vi "Multi-camera acquisition of images.vi"() -> ()   [LabVIEW 2009]
uses:
  D/Program Files (x86)/National Instruments/LabVIEW 2015/user.lib/LabViewDVPCamera/LabViewDVPCamera.lvlib
panel:
  out "new picture 4":picture caption="新图片"
  in  "CloseFlg 4":i32
  in  "CameraList 4":u16(ring) caption="CameraList" items=["USB2_1.2M_MONO(39)@UE121000027", "USB2_3M(19)@1112121"]
  in  "Set 4":bool
  in  "Open 4":bool
  in  "Close 4":bool
  in  "ScanCamera 4":bool
  out "handle 4":u32
  out "new picture 3":picture caption="新图片"
  in  "CloseFlg 3":i32
  in  "CameraList 3":u16(ring) caption="CameraList" items=["USB2_1.2M_MONO(39)@UE121000027", "USB2_3M(19)@1112121"]
  in  "Set 3":bool
  in  "Open 3":bool
  in  "Close 3":bool
  in  "ScanCamera 3":bool
  out "handle 3":u32
  out "new picture 2":picture caption="新图片"
  in  "CloseFlg 2":i32
  in  "CameraList 2":u16(ring) caption="CameraList" items=["USB2_1.2M_MONO(39)@UE121000027", "USB2_3M(19)@1112121"]
  in  "Set 2":bool
  in  "Open 2":bool
  in  "Close 2":bool
  in  "ScanCamera 2":bool
  out "handle 2":u32
  out "new picture":picture caption="新图片"
  in  "CloseFlg":i32
  in  "CameraList":u16(ring) items=["USB2_1.2M_MONO(39)@UE121000027", "USB2_3M(19)@1112121"]
  in  "Set":bool
  in  "Open":bool
  in  "Close":bool
  in  "ScanCamera":bool
  out "handle":u32
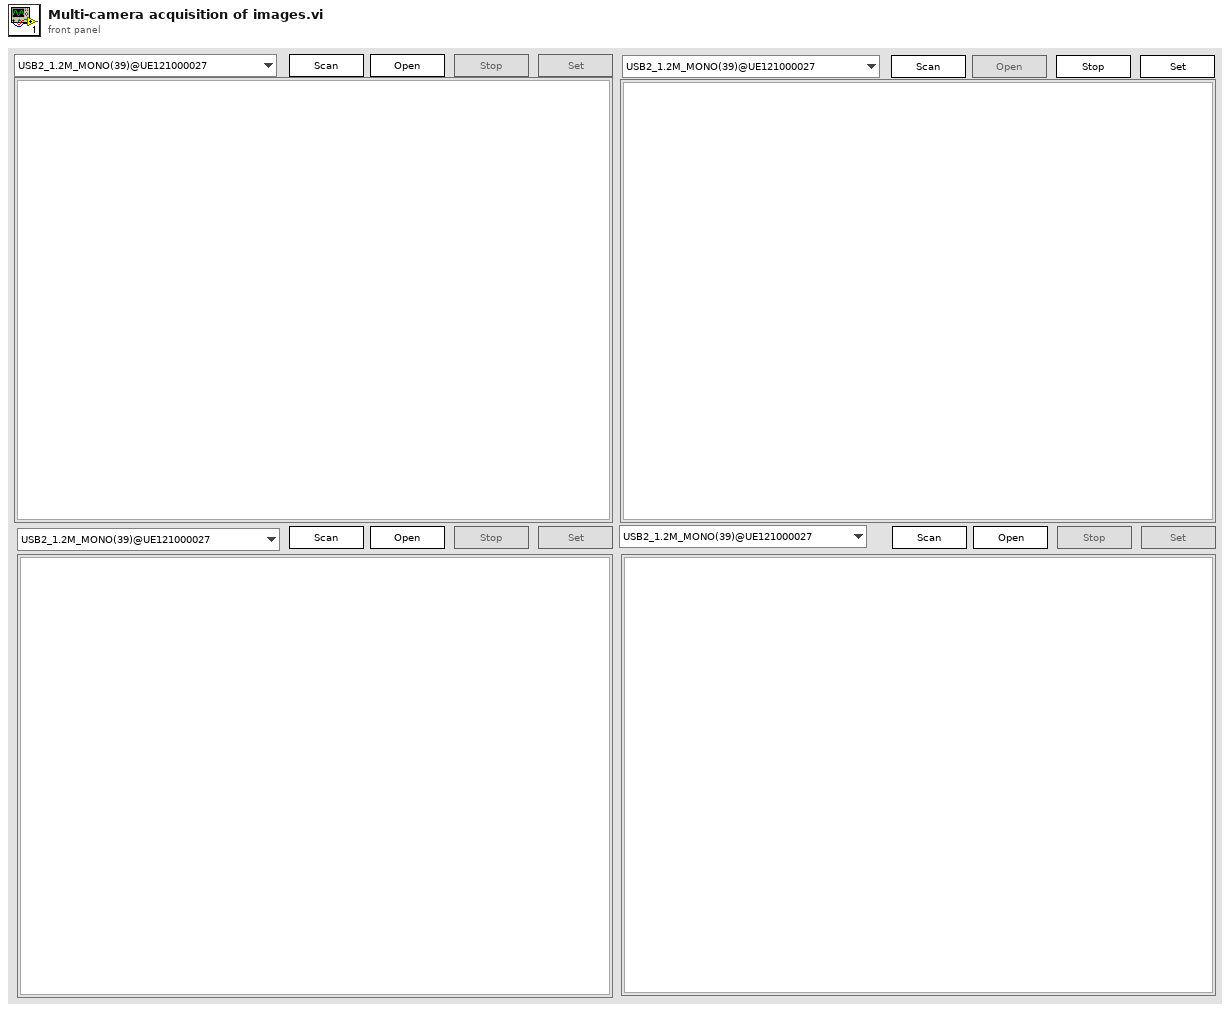
[diagram p1: front panel]
types:
  T1 = enum8{"Enabled", "Disabled", "Disabled and Grayed Out"}
  T2 = typedef "LVStringsAndValuesArrayTypeDef_U16.ctl" = cluster{"String":string, "Value":u16}[]
  T3 = cluster{"image type":i16, "image depth":u8, u8[], "无符号8位数组":u8[], u32[], cluster{u16, u16, u16, u16}}
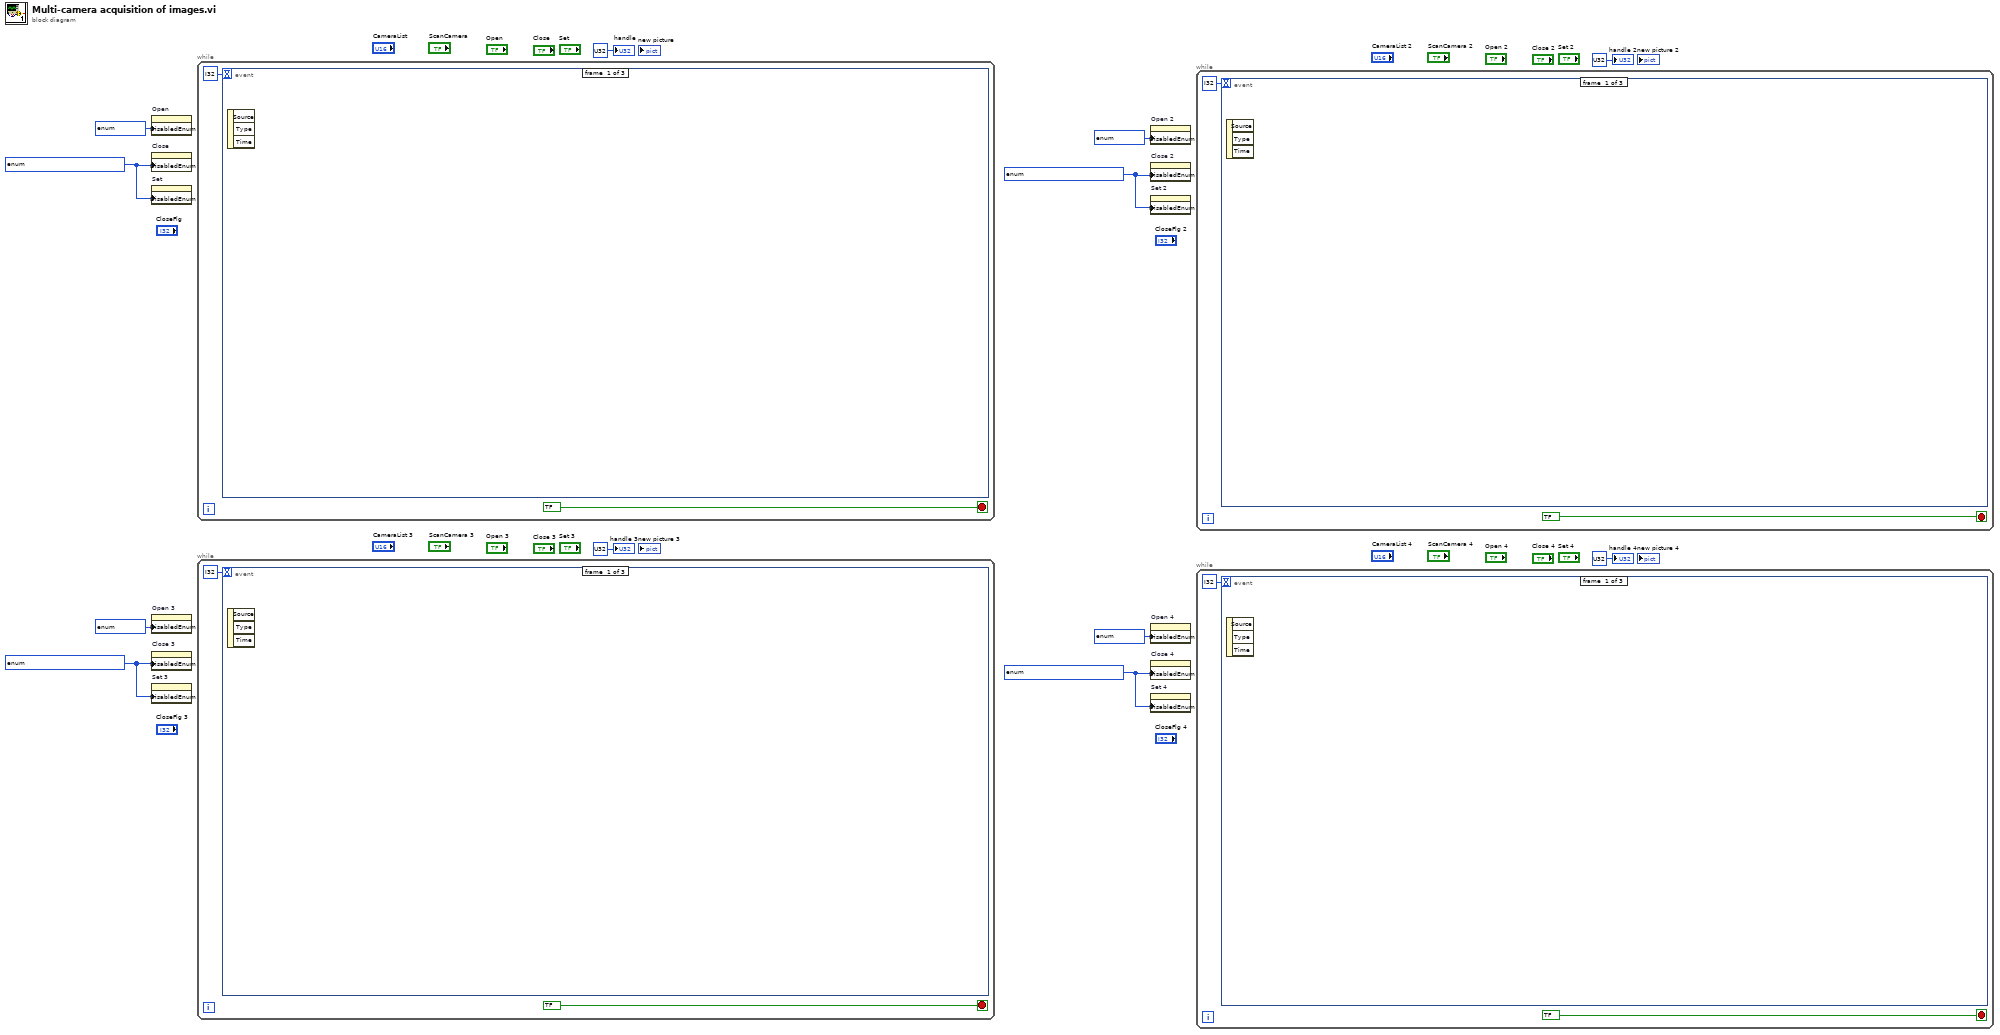
[diagram p0: block diagram]
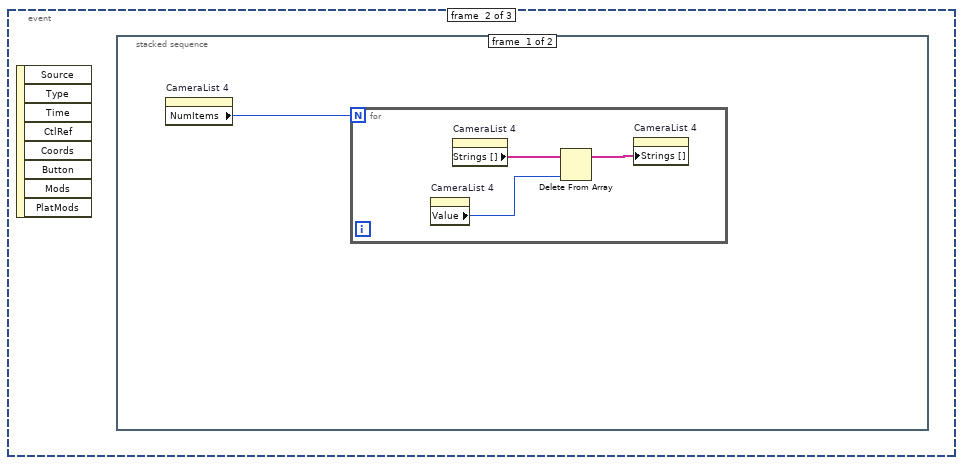
[diagram p2: hidden frame]
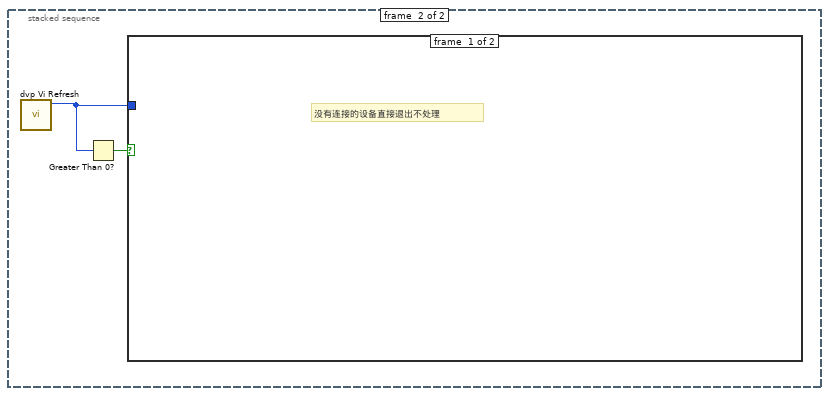
[diagram p3: hidden frame]
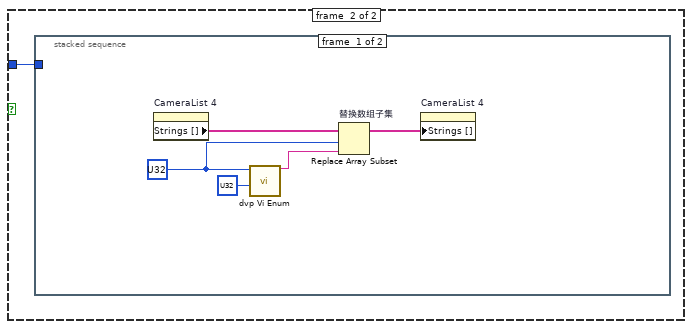
[diagram p4: hidden frame]
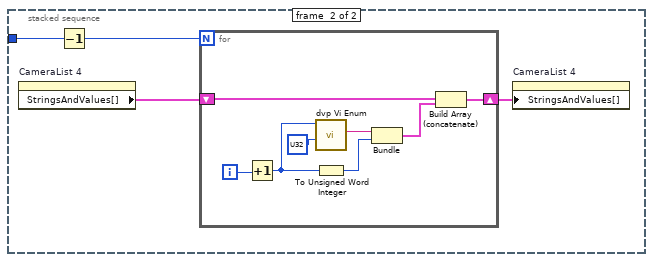
[diagram p5: hidden frame]
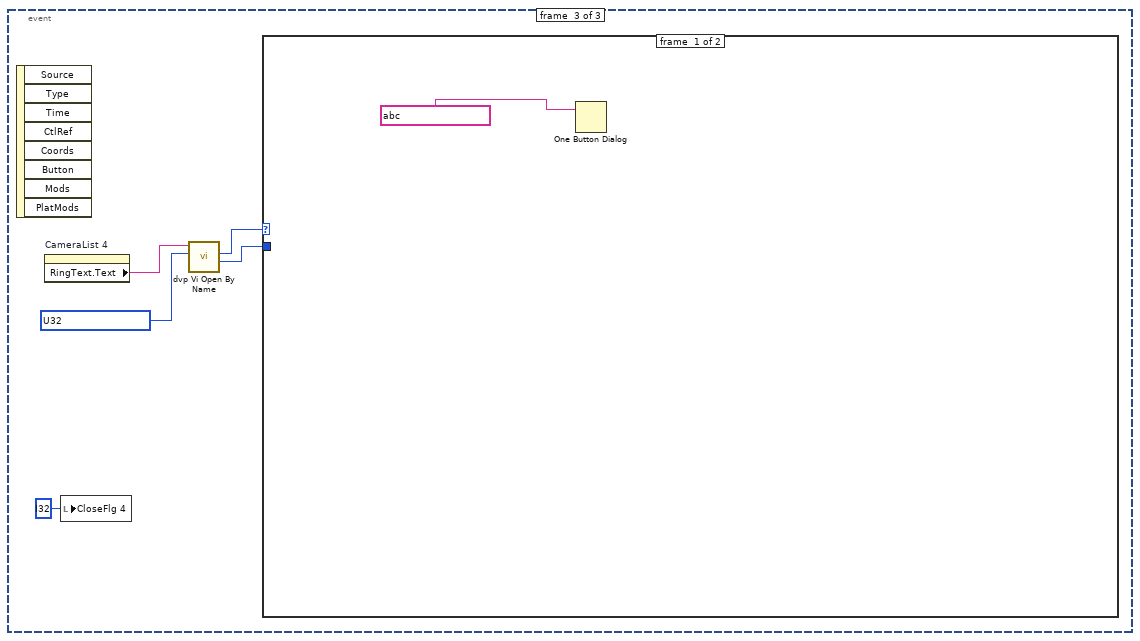
[diagram p6: hidden frame]
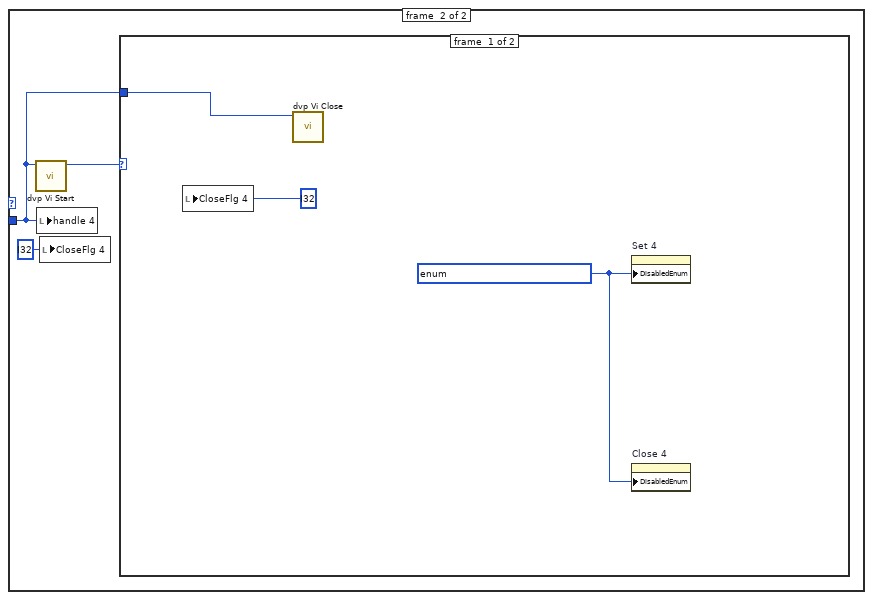
[diagram p7: hidden frame]
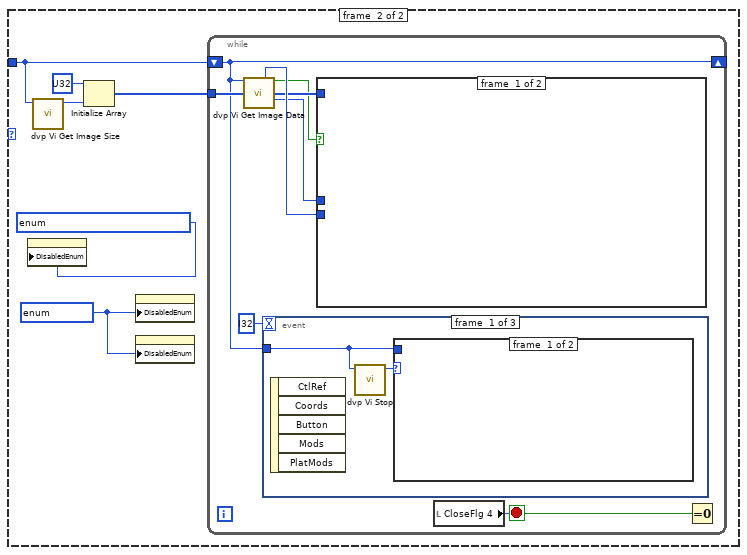
[diagram p8: hidden frame]
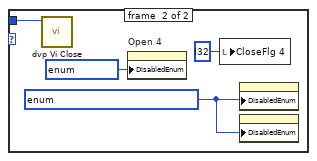
[diagram p9: hidden frame]
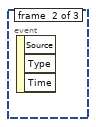
[diagram p10: hidden frame]
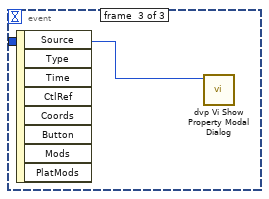
[diagram p11: hidden frame]
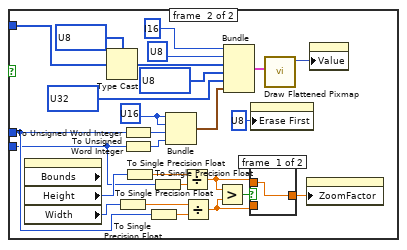
[diagram p12: hidden frame]
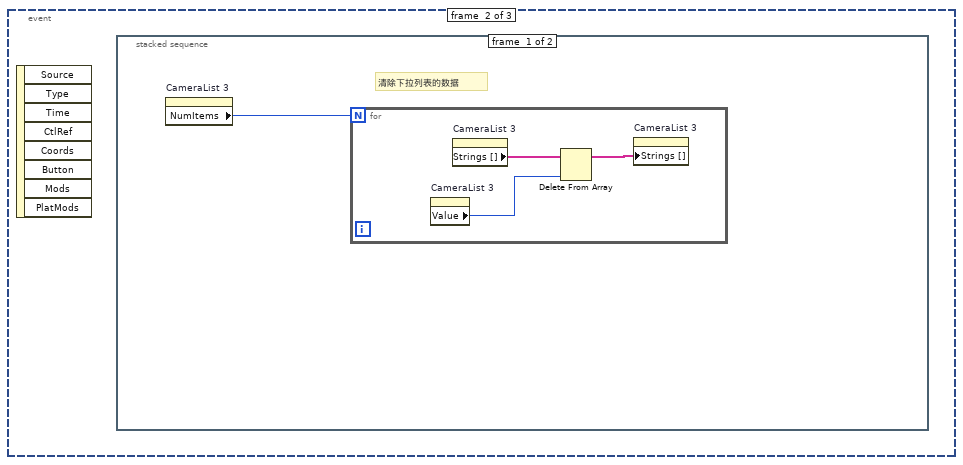
[diagram p14: hidden frame]
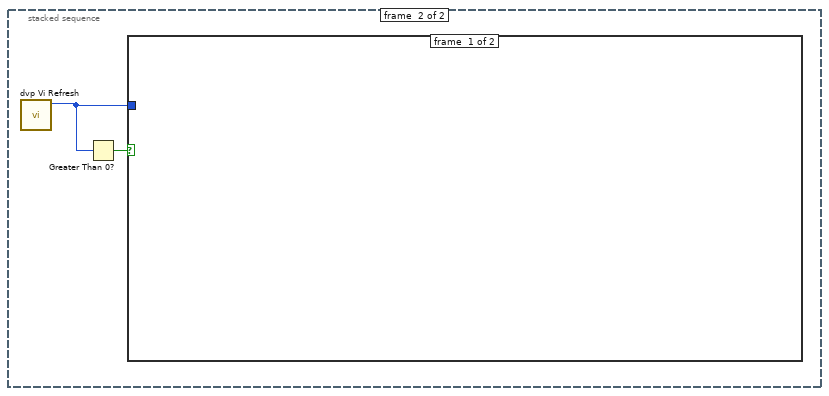
[diagram p15: hidden frame]
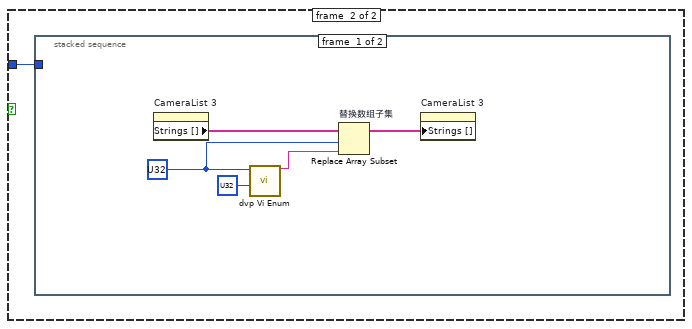
[diagram p16: hidden frame]
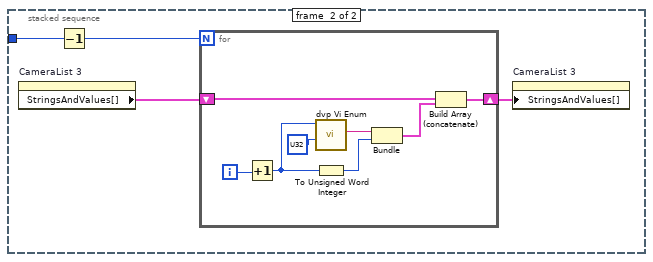
[diagram p17: hidden frame]
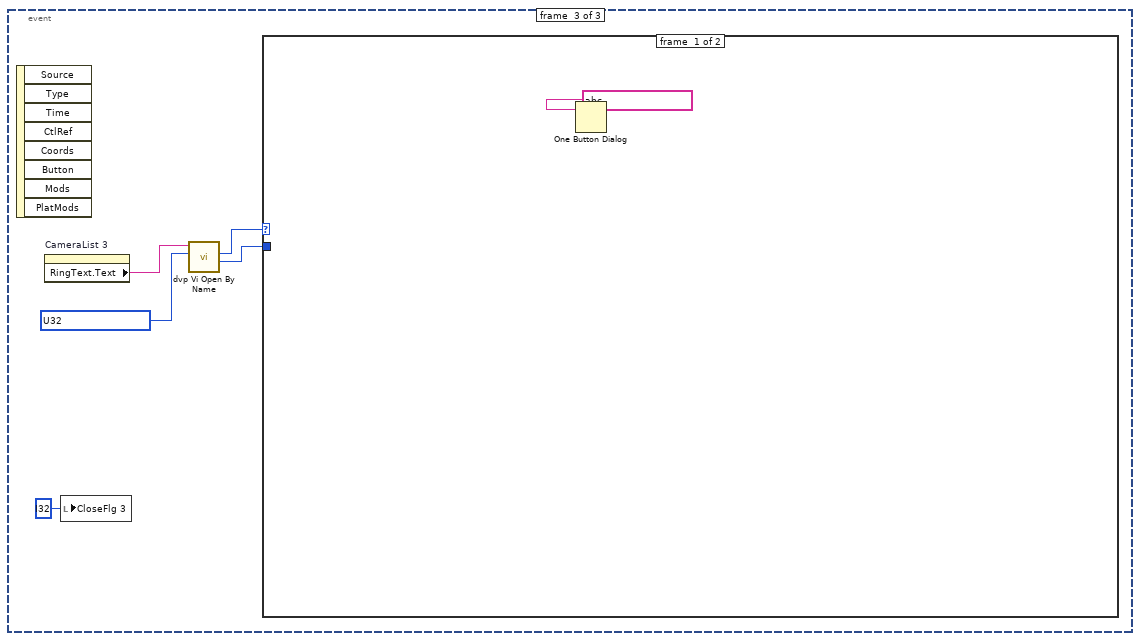
[diagram p18: hidden frame]
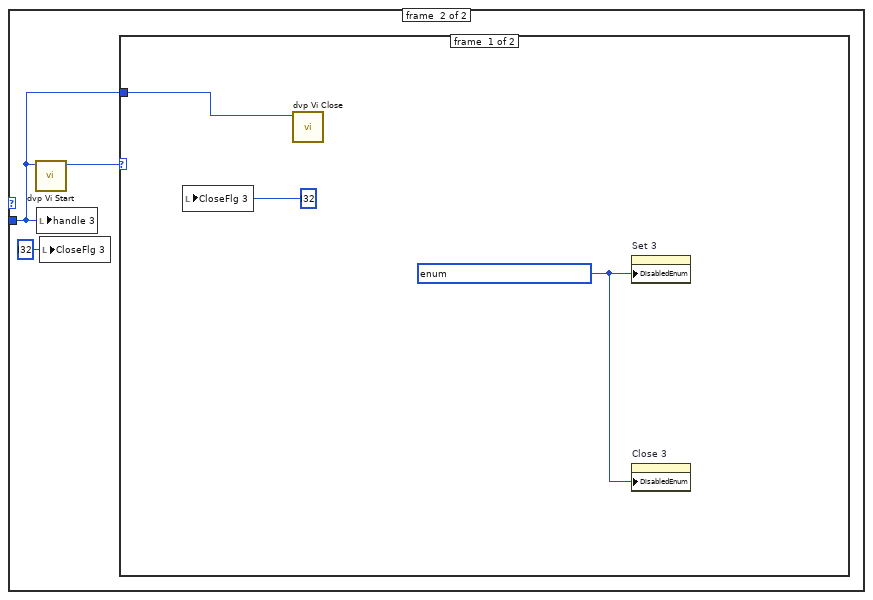
[diagram p19: hidden frame]
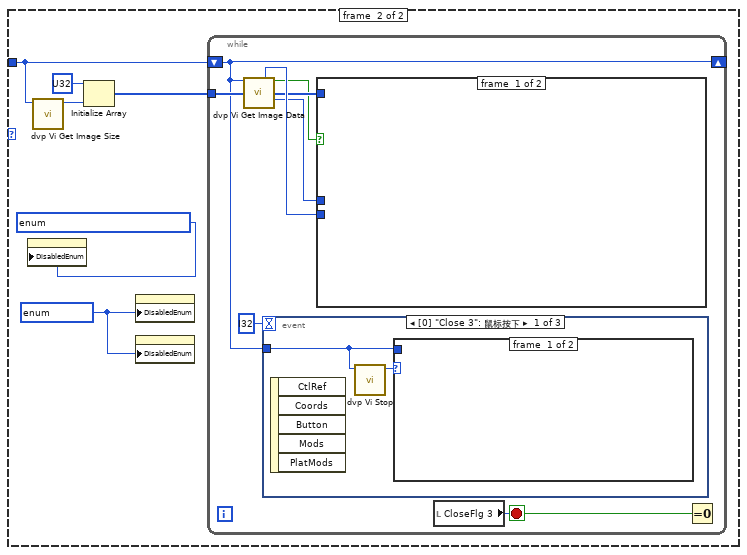
[diagram p20: hidden frame]
diagram:
  w2 = T1 ? ("禁用")
  w5 = T1 ? ("禁用")
  w8 = T1 ? ("禁用")
  w11 = T1 ? ("禁用")
  n1 = property on="Open" class="Bool"("DisabledEnum"=T1 ? ("禁用")) -> ()  [unwired: 2 in, 2 out]
  n2 = property on="Close" class="Bool"("DisabledEnum"=w11) -> ()  [unwired: 2 in, 2 out]
  n3 = property on="Set" class="Bool"("DisabledEnum"=w11) -> ()  [unwired: 2 in, 2 out]
  n4 = property on="Open 3" class="Bool"("DisabledEnum"=T1 ? ("禁用")) -> ()  [unwired: 2 in, 2 out]
  n5 = property on="Close 3" class="Bool"("DisabledEnum"=w5) -> ()  [unwired: 2 in, 2 out]
  n6 = property on="Set 3" class="Bool"("DisabledEnum"=w5) -> ()  [unwired: 2 in, 2 out]
  n7 = while {
    stop <- bool ? stop-if-true
    n8 = event shown="[2] \"Open\": 鼠标按下" {
      selector: _ -> [_ _ _]
      dyn-events: _ -> [_ _ _]
      timeout: i32 ? -> [_ _ _]
      event #0 {
        n9 = event-data() -> ()  [unwired: 1 in, 3 out]
      }
      event #1 {
        n10 = event-data() -> ()  [unwired: 1 in, 8 out]
        n11 = stacked-sequence "清除下拉列表的数据" {
          frame #0 {
            n12 = property on="CameraList" class="Ring (严格)"() -> ("NumItems"=w15:u32)  [unwired: 2 in, 2 out]
            n13 = for {
              N: w15 -> [_]
              n14 = property on="CameraList" class="Ring (严格)"() -> ("Value"=w17:u16)  [unwired: 2 in, 2 out]
              n15 = property on="CameraList" class="Ring (严格)"() -> ("Strings []"=w16:string[])  [unwired: 2 in, 2 out]
              n16 = Delete From Array ("删除数组元素")(array=w16, index=w17) -> (array with subset deleted=w18:string[])  [unwired: 1 in, 1 out]
              n17 = property on="CameraList" class="Ring (严格)"("Strings []"=w18) -> ()  [unwired: 2 in, 2 out]
            }
          }
          frame #1 {
            n18 = call "dvp Vi Refresh.vi"() -> ("pCount out"=w20:u32)  [unwired: 10 in, 1 out]
            n19 = Greater Than 0?(x=w20) -> (x > 0?=w19:bool)
            n20 = case shown="真" w19 {
              tunnel: w20 -> [_ w21]
              frame #0 {
              }
              frame #1 {
                n21 = stacked-sequence {
                  tunnel: w21 -> [_ w28]
                  frame #0 {
                    w22 = u32 ? ("index")
                    n22 = property on="CameraList" class="Ring (严格)"() -> ("Strings []"=w25:string[])  [unwired: 2 in, 2 out]
                    n23 = call "dvp Vi Enum.vi"("unSize"=u32 ?, "index"=w22) -> ("friendlyName out"=w24:string)  [unwired: 8 in, 1 out]
                    n24 = Replace Array Subset "替换数组子集"(array=w25, new element=w24, index=w22) -> (w26:string[])
                    n25 = property on="CameraList" class="Ring (严格)"("Strings []"=w26) -> ()  [unwired: 2 in, 2 out]
                  }
                  frame #1 {
                    n26 = property on="CameraList" class="Ring (严格)"() -> ("StringsAndValues[]"=w30:T2)  [unwired: 2 in, 2 out]
                    n27 = Decrement(x=w28) -> (x-1=w27:u32)
                    n28 = for {
                      N: w27 -> [_]
                      shift-right: [w37] -> w29
                      shift-left: w30 -> [w35]
                      i -> [w32]
                      n29 = Increment(x=w32) -> (x+1=w31:i32)
                      n30 = call "dvp Vi Enum.vi"("unSize"=u32 ?, "index"=w31) -> ("friendlyName out"=w38:string)  [unwired: 8 in, 1 out]
                      n31 = To Unsigned Word Integer(number=w31) -> (unsigned 16bit integer=w34:u16)
                      n32 = Bundle("friendlyName out"=w38, w34) -> (w36:cluster{"friendlyName out":string, u16})  [unwired: 1 in]
                      n33 = Build Array (concatenate)(w35, w36) -> (w37:T2)
                    }
                    n34 = property on="CameraList" class="Ring (严格)"("StringsAndValues[]"=w29) -> ()  [unwired: 2 in, 2 out]
                  }
                }
              }
            }
          }
        }
      }
      event #2 {
        w41 = u32 ? items=["OPEN_OFFLINE", "OPEN_NORMAL"] ("type")
        n35 = event-data() -> ()  [unwired: 1 in, 8 out]
        n36 = property on="CameraList" class="Ring (严格)"() -> ("RingText.Text"=w40:string)  [unwired: 2 in, 2 out]
        n37 = local write "CloseFlg"(i32 ? ("CloseFlg")) -> ()
        n38 = call "dvp Vi Open By Name.vi"("type"=w41, "friendlyName"=w40) -> ("pHandle out"=w43:u32, "function return"=w42:u32)  [unwired: 7 in, 1 out]
        n39 = case shown="1" w42 {
          tunnel: w43 -> [_ w47]
          frame #0 {
            n40 = One Button Dialog(message=string ? ("消息")) -> ()  [unwired: 1 in, 1 out]
          }
          frame #1 {
            n41 = call "dvp Vi Start.vi"("handle"=w47) -> ("function return"=w45:u32)  [unwired: 10 in]
            n42 = local write "handle"(w47) -> ()
            n43 = local write "CloseFlg"(i32 ? ("CloseFlg")) -> ()
            n44 = case shown="1" w45 {
              tunnel: w47 -> [w50 w52]
              frame #0 {
                w49 = T1 ? ("禁用")
                n45 = local write "CloseFlg"(i32 ? ("CloseFlg")) -> ()
                n46 = call "dvp Vi Close.vi"("handle"=w50) -> ()  [unwired: 10 in, 1 out]
                n47 = property on="Set" class="Bool"("DisabledEnum"=w49) -> ()  [unwired: 2 in, 2 out]
                n48 = property on="Close" class="Bool"("DisabledEnum"=w49) -> ()  [unwired: 2 in, 2 out]
              }
              frame #1 {
                w56 = T1 ? ("禁用")
                n49 = property on="Open" class="Bool"("DisabledEnum"=T1 ? ("禁用")) -> ()  [unwired: 2 in, 2 out]
                n50 = call "dvp Vi Get Image Size.vi"("handle"=w52) -> ("function return"=w51:u32)  [unwired: 10 in]
                n51 = Initialize Array(u32 ? ("元素"), w51) -> (w53:u32[])
                n52 = property on="Set" class="Bool"("DisabledEnum"=w56) -> ()  [unwired: 2 in, 2 out]
                n53 = property on="Close" class="Bool"("DisabledEnum"=w56) -> ()  [unwired: 2 in, 2 out]
                n54 = while {
                  shift-right: [w61] -> _
                  shift-left: w52 -> [w61]
                  tunnel: w53 -> [w62]
                  stop <- w64 stop-if-true
                  n55 = call "dvp Vi Get Image Data.vi"("handle"=w61, "pbuffer"=w62) -> ("piHeight out"=w60:i32, "function return"=w57:bool, "pbuffer out"=w58:u32[], "piWidth out"=w59:i32)  [unwired: 9 in, 1 out]
                  n56 = event shown="[0] \"Close\": 鼠标按下" {
                    selector: _ -> [_ _ _]
                    dyn-events: _ -> [_ _ _]
                    timeout: i32 ? -> [_ _ _]
                    tunnel: w61 -> [w66 _ w72]
                    event #0 {
                      n57 = event-data() -> ()  [unwired: 1 in, 5 out]
                      n58 = call "dvp Vi Stop.vi"("handle"=w66) -> ("function return"=w67:u32)  [unwired: 10 in]
                      n59 = case shown="1" w67 {
                        tunnel: w66 -> [_ w69]
                        frame #0 {
                        }
                        frame #1 {
                          w68 = T1 ? ("禁用")
                          n60 = call "dvp Vi Close.vi"("handle"=w69) -> ()  [unwired: 10 in, 1 out]
                          n61 = property on="Open" class="Bool"("DisabledEnum"=T1 ? ("禁用")) -> ()  [unwired: 2 in, 2 out]
                          n62 = local write "CloseFlg"(i32 ? ("CloseFlg")) -> ()
                          n63 = property on="Close" class="Bool"("DisabledEnum"=w68) -> ()  [unwired: 2 in, 2 out]
                          n64 = property on="Set" class="Bool"("DisabledEnum"=w68) -> ()  [unwired: 2 in, 2 out]
                        }
                      }
                    }
                    event #1 {
                      n65 = event-data() -> ()  [unwired: 1 in, 3 out]
                    }
                    event #2 {
                      n66 = event-data() -> ()  [unwired: 1 in, 8 out]
                      n67 = call "dvp Vi Show Property Modal Dialog.vi"("handle"=w72) -> ()  [unwired: 10 in, 1 out]
                    }
                  }
                  n68 = case shown="真" w57 {
                    tunnel: w58 -> [_ w76]
                    tunnel: w59 -> [_ w80]
                    tunnel: w60 -> [_ w79]
                    frame #0 {
                    }
                    frame #1 {
                      w96 = u16 ?
                      n69 = property on="new picture" class="Pict" props=[]() -> ("Height"=w89:u32, "Width"=w88:u32)  [unwired: 2 in, 3 out]
                      n70 = Type Cast(type=u8[] ?, x=w76) -> (*(type *) &x=w75:u8[])
                      n71 = To Single Precision Float(number=w88) -> (single precision float=w81:sgl)
                      n72 = To Unsigned Word Integer(number=w80) -> (unsigned 16bit integer=w95:u16)
                      n73 = To Unsigned Word Integer(number=w79) -> (unsigned 16bit integer=w94:u16)
                      n74 = To Single Precision Float(number=w89) -> (single precision float=w87:sgl)
                      n75 = To Single Precision Float(number=w80) -> (single precision float=w85:sgl)
                      n76 = To Single Precision Float(number=w79) -> (single precision float=w86:sgl)
                      n77 = Bundle ("图像尺寸")(w96, w96, w95, w94) -> (w93:cluster{u16, u16, u16, u16})  [unwired: 1 in]
                      n78 = Divide(x=w87, y=w86) -> (x/y=w83:sgl)
                      n79 = Divide(x=w81, y=w85) -> (x/y=w82:sgl)
                      n80 = Greater?(x=w83, y=w82) -> (0:w84:bool)
                      n81 = Bundle ("图像数据")("image type"=i16 ?, "image depth"=u8 ?, w75, "无符号8位数组"=u8[] ?, u32[] ?, w93) -> (w77:T3)  [unwired: 1 in]
                      n82 = case shown="真" w84 {
                        tunnel: w83 -> [w99 _]
                        tunnel: w82 -> [_ w100]
                        tunnel: [w99 w100] -> w78
                        frame #0 {
                        }
                        frame #1 {
                        }
                      }
                      n83 = property on="new picture" class="Pict"("Erase First"=u8 ? ("画前清除图片")) -> ()  [unwired: 2 in, 2 out]
                      n84 = call <vilib>:"Draw Flattened Pixmap.vi"("image data"=w77) -> ("new picture"=w90:picture)  [unwired: 8 in]
                      n85 = property on="new picture" class="Pict"("ZoomFactor"=w78) -> ()  [unwired: 2 in, 2 out]
                      n86 = property on="new picture" class="Pict"("Value"=w90) -> ()  [unwired: 2 in, 2 out]
                    }
                  }
                  n87 = local read "CloseFlg"() -> (w63:i32)
                  n88 = Equal To 0?(x=w63) -> (x = 0?=w64:bool)
                }
              }
            }
          }
        }
      }
    }
  }
  n89 = while {
    stop <- bool ? stop-if-true
    n90 = event shown="[2] \"Open 3\": 鼠标按下" {
      selector: _ -> [_ _ _]
      dyn-events: _ -> [_ _ _]
      timeout: i32 ? -> [_ _ _]
      event #0 {
        n91 = event-data() -> ()  [unwired: 1 in, 3 out]
      }
      event #1 {
        n92 = event-data() -> ()  [unwired: 1 in, 8 out]
        n93 = stacked-sequence "清除下拉列表的数据" {
          frame #0 {
            # "清除下拉列表的数据"
            n94 = property on="CameraList 3" class="Ring (严格)"() -> ("NumItems"=w103:u32)  [unwired: 2 in, 2 out]
            n95 = for {
              N: w103 -> [_]
              n96 = property on="CameraList 3" class="Ring (严格)"() -> ("Value"=w105:u16)  [unwired: 2 in, 2 out]
              n97 = property on="CameraList 3" class="Ring (严格)"() -> ("Strings []"=w104:string[])  [unwired: 2 in, 2 out]
              n98 = Delete From Array ("删除数组元素")(array=w104, index=w105) -> (array with subset deleted=w106:string[])  [unwired: 1 in, 1 out]
              n99 = property on="CameraList 3" class="Ring (严格)"("Strings []"=w106) -> ()  [unwired: 2 in, 2 out]
            }
          }
          frame #1 {
            n100 = call "dvp Vi Refresh.vi"() -> ("pCount out"=w108:u32)  [unwired: 10 in, 1 out]
            n101 = Greater Than 0?(x=w108) -> (x > 0?=w107:bool)
            n102 = case shown="真" w107 {
              tunnel: w108 -> [_ w109]
              frame #0 {
              }
              frame #1 {
                n103 = stacked-sequence {
                  tunnel: w109 -> [_ w116]
                  frame #0 {
                    w110 = u32 ? ("index")
                    n104 = property on="CameraList 3" class="Ring (严格)"() -> ("Strings []"=w113:string[])  [unwired: 2 in, 2 out]
                    n105 = call "dvp Vi Enum.vi"("unSize"=u32 ?, "index"=w110) -> ("friendlyName out"=w112:string)  [unwired: 8 in, 1 out]
                    n106 = Replace Array Subset "替换数组子集"(array=w113, new element=w112, index=w110) -> (w114:string[])
                    n107 = property on="CameraList 3" class="Ring (严格)"("Strings []"=w114) -> ()  [unwired: 2 in, 2 out]
                  }
                  frame #1 {
                    n108 = property on="CameraList 3" class="Ring (严格)"() -> ("StringsAndValues[]"=w118:T2)  [unwired: 2 in, 2 out]
                    n109 = Decrement(x=w116) -> (x-1=w115:u32)
                    n110 = for {
                      N: w115 -> [_]
                      shift-right: [w125] -> w117
                      shift-left: w118 -> [w123]
                      i -> [w120]
                      n111 = Increment(x=w120) -> (x+1=w119:i32)
                      n112 = call "dvp Vi Enum.vi"("unSize"=u32 ?, "index"=w119) -> ("friendlyName out"=w126:string)  [unwired: 8 in, 1 out]
                      n113 = To Unsigned Word Integer(number=w119) -> (unsigned 16bit integer=w122:u16)
                      n114 = Bundle("friendlyName out"=w126, w122) -> (w124:cluster{"friendlyName out":string, u16})  [unwired: 1 in]
                      n115 = Build Array (concatenate)(w123, w124) -> (w125:T2)
                    }
                    n116 = property on="CameraList 3" class="Ring (严格)"("StringsAndValues[]"=w117) -> ()  [unwired: 2 in, 2 out]
                  }
                }
              }
            }
          }
        }
      }
      event #2 {
        w129 = u32 ? items=["OPEN_OFFLINE", "OPEN_NORMAL"] ("type")
        n117 = event-data() -> ()  [unwired: 1 in, 8 out]
        n118 = property on="CameraList 3" class="Ring (严格)"() -> ("RingText.Text"=w128:string)  [unwired: 2 in, 2 out]
        n119 = local write "CloseFlg 3"(i32 ? ("CloseFlg")) -> ()
        n120 = call "dvp Vi Open By Name.vi"("type"=w129, "friendlyName"=w128) -> ("pHandle out"=w131:u32, "function return"=w130:u32)  [unwired: 7 in, 1 out]
        n121 = case shown="1" w130 {
          tunnel: w131 -> [_ w135]
          frame #0 {
            n122 = One Button Dialog(message=string ? ("消息")) -> ()  [unwired: 1 in, 1 out]
          }
          frame #1 {
            n123 = call "dvp Vi Start.vi"("handle"=w135) -> ("function return"=w133:u32)  [unwired: 10 in]
            n124 = local write "handle 3"(w135) -> ()
            n125 = local write "CloseFlg 3"(i32 ? ("CloseFlg")) -> ()
            n126 = case shown="1" w133 {
              tunnel: w135 -> [w138 w140]
              frame #0 {
                w137 = T1 ? ("禁用")
                n127 = local write "CloseFlg 3"(i32 ? ("CloseFlg")) -> ()
                n128 = call "dvp Vi Close.vi"("handle"=w138) -> ()  [unwired: 10 in, 1 out]
                n129 = property on="Set 3" class="Bool"("DisabledEnum"=w137) -> ()  [unwired: 2 in, 2 out]
                n130 = property on="Close 3" class="Bool"("DisabledEnum"=w137) -> ()  [unwired: 2 in, 2 out]
              }
              frame #1 {
                w144 = T1 ? ("禁用")
                n131 = property on="Open 3" class="Bool"("DisabledEnum"=T1 ? ("禁用")) -> ()  [unwired: 2 in, 2 out]
                n132 = call "dvp Vi Get Image Size.vi"("handle"=w140) -> ("function return"=w139:u32)  [unwired: 10 in]
                n133 = Initialize Array(u32 ? ("元素"), w139) -> (w141:u32[])
                n134 = property on="Set 3" class="Bool"("DisabledEnum"=w144) -> ()  [unwired: 2 in, 2 out]
                n135 = property on="Close 3" class="Bool"("DisabledEnum"=w144) -> ()  [unwired: 2 in, 2 out]
                n136 = while {
                  shift-right: [w149] -> _
                  shift-left: w140 -> [w149]
                  tunnel: w141 -> [w150]
                  stop <- w152 stop-if-true
                  n137 = call "dvp Vi Get Image Data.vi"("handle"=w149, "pbuffer"=w150) -> ("piHeight out"=w148:i32, "function return"=w145:bool, "pbuffer out"=w146:u32[], "piWidth out"=w147:i32)  [unwired: 9 in, 1 out]
                  n138 = event shown="[0] \"Close 3\": 鼠标按下" {
                    selector: _ -> [_ _ _]
                    dyn-events: _ -> [_ _ _]
                    timeout: i32 ? -> [_ _ _]
                    tunnel: w149 -> [w154 _ w160]
                    event #0 {
                      n139 = event-data() -> ()  [unwired: 1 in, 5 out]
                      n140 = call "dvp Vi Stop.vi"("handle"=w154) -> ("function return"=w155:u32)  [unwired: 10 in]
                      n141 = case shown="1" w155 {
                        tunnel: w154 -> [_ w157]
                        frame #0 {
                        }
                        frame #1 {
                          w156 = T1 ? ("禁用")
                          n142 = call "dvp Vi Close.vi"("handle"=w157) -> ()  [unwired: 10 in, 1 out]
                          n143 = property on="Open 3" class="Bool"("DisabledEnum"=T1 ? ("禁用")) -> ()  [unwired: 2 in, 2 out]
                          n144 = local write "CloseFlg 3"(i32 ? ("CloseFlg")) -> ()
                          n145 = property on="Close 3" class="Bool"("DisabledEnum"=w156) -> ()  [unwired: 2 in, 2 out]
                          n146 = property on="Set 3" class="Bool"("DisabledEnum"=w156) -> ()  [unwired: 2 in, 2 out]
                        }
                      }
                    }
                    event #1 {
                      n147 = event-data() -> ()  [unwired: 1 in, 3 out]
                    }
                    event #2 {
                      n148 = event-data() -> ()  [unwired: 1 in, 8 out]
                      n149 = call "dvp Vi Show Property Modal Dialog.vi"("handle"=w160) -> ()  [unwired: 10 in, 1 out]
                    }
                  }
                  n150 = case shown="真" w145 {
                    tunnel: w146 -> [_ w164]
                    tunnel: w147 -> [_ w168]
                    tunnel: w148 -> [_ w167]
                    frame #0 {
                    }
                    frame #1 {
                      w184 = u16 ?
                      n151 = property on="new picture 3" class="Pict" props=[]() -> ("Height"=w177:u32, "Width"=w176:u32)  [unwired: 2 in, 3 out]
                      n152 = Type Cast(type=u8[] ?, x=w164) -> (*(type *) &x=w163:u8[])
                      n153 = To Single Precision Float(number=w176) -> (single precision float=w169:sgl)
                      n154 = To Unsigned Word Integer(number=w168) -> (unsigned 16bit integer=w183:u16)
                      n155 = To Unsigned Word Integer(number=w167) -> (unsigned 16bit integer=w182:u16)
                      n156 = To Single Precision Float(number=w177) -> (single precision float=w175:sgl)
                      n157 = To Single Precision Float(number=w168) -> (single precision float=w173:sgl)
                      n158 = To Single Precision Float(number=w167) -> (single precision float=w174:sgl)
                      n159 = Bundle ("图像尺寸")(w184, w184, w183, w182) -> (w181:cluster{u16, u16, u16, u16})  [unwired: 1 in]
                      n160 = Divide(x=w175, y=w174) -> (x/y=w171:sgl)
                      n161 = Divide(x=w169, y=w173) -> (x/y=w170:sgl)
                      n162 = Greater?(x=w171, y=w170) -> (0:w172:bool)
                      n163 = Bundle ("图像数据")("image type"=i16 ?, "image depth"=u8 ?, w163, "无符号8位数组"=u8[] ?, u32[] ?, w181) -> (w165:T3)  [unwired: 1 in]
                      n164 = case shown="真" w172 {
                        tunnel: w171 -> [w187 _]
                        tunnel: w170 -> [_ w188]
                        tunnel: [w187 w188] -> w166
                        frame #0 {
                        }
                        frame #1 {
                        }
                      }
                      n165 = property on="new picture 3" class="Pict"("Erase First"=u8 ? ("画前清除图片")) -> ()  [unwired: 2 in, 2 out]
                      n166 = call <vilib>:"Draw Flattened Pixmap.vi"("image data"=w165) -> ("new picture"=w178:picture)  [unwired: 8 in]
                      n167 = property on="new picture 3" class="Pict"("ZoomFactor"=w166) -> ()  [unwired: 2 in, 2 out]
                      n168 = property on="new picture 3" class="Pict"("Value"=w178) -> ()  [unwired: 2 in, 2 out]
                    }
                  }
                  n169 = local read "CloseFlg 3"() -> (w151:i32)
                  n170 = Equal To 0?(x=w151) -> (x = 0?=w152:bool)
                }
              }
            }
          }
        }
      }
    }
  }
  n171 = property on="Open 2" class="Bool"("DisabledEnum"=T1 ? ("禁用")) -> ()  [unwired: 2 in, 2 out]
  n172 = property on="Close 2" class="Bool"("DisabledEnum"=w8) -> ()  [unwired: 2 in, 2 out]
  n173 = property on="Set 2" class="Bool"("DisabledEnum"=w8) -> ()  [unwired: 2 in, 2 out]
  n174 = property on="Open 4" class="Bool"("DisabledEnum"=T1 ? ("禁用")) -> ()  [unwired: 2 in, 2 out]
  n175 = property on="Close 4" class="Bool"("DisabledEnum"=w2) -> ()  [unwired: 2 in, 2 out]
  n176 = property on="Set 4" class="Bool"("DisabledEnum"=w2) -> ()  [unwired: 2 in, 2 out]
  n177 = while {
    stop <- bool ? stop-if-true
    n178 = event shown="[2] \"Open 2\": 鼠标按下" {
      selector: _ -> [_ _ _]
      dyn-events: _ -> [_ _ _]
      timeout: i32 ? -> [_ _ _]
      event #0 {
        n179 = event-data() -> ()  [unwired: 1 in, 3 out]
      }
      event #1 {
        n180 = event-data() -> ()  [unwired: 1 in, 8 out]
        n181 = stacked-sequence "清除下拉列表的数据" {
          frame #0 {
            n182 = property on="CameraList 2" class="Ring (严格)"() -> ("NumItems"=w191:u32)  [unwired: 2 in, 2 out]
            n183 = for {
              N: w191 -> [_]
              n184 = property on="CameraList 2" class="Ring (严格)"() -> ("Value"=w193:u16)  [unwired: 2 in, 2 out]
              n185 = property on="CameraList 2" class="Ring (严格)"() -> ("Strings []"=w192:string[])  [unwired: 2 in, 2 out]
              n186 = Delete From Array ("删除数组元素")(array=w192, index=w193) -> (array with subset deleted=w194:string[])  [unwired: 1 in, 1 out]
              n187 = property on="CameraList 2" class="Ring (严格)"("Strings []"=w194) -> ()  [unwired: 2 in, 2 out]
            }
          }
          frame #1 {
            n188 = call "dvp Vi Refresh.vi"() -> ("pCount out"=w196:u32)  [unwired: 10 in, 1 out]
            n189 = Greater Than 0?(x=w196) -> (x > 0?=w195:bool)
            n190 = case shown="真" w195 {
              tunnel: w196 -> [_ w197]
              frame #0 {
              }
              frame #1 {
                n191 = stacked-sequence {
                  tunnel: w197 -> [_ w204]
                  frame #0 {
                    w198 = u32 ? ("index")
                    n192 = property on="CameraList 2" class="Ring (严格)"() -> ("Strings []"=w201:string[])  [unwired: 2 in, 2 out]
                    n193 = call "dvp Vi Enum.vi"("unSize"=u32 ?, "index"=w198) -> ("friendlyName out"=w200:string)  [unwired: 8 in, 1 out]
                    n194 = Replace Array Subset "替换数组子集"(array=w201, new element=w200, index=w198) -> (w202:string[])
                    n195 = property on="CameraList 2" class="Ring (严格)"("Strings []"=w202) -> ()  [unwired: 2 in, 2 out]
                  }
                  frame #1 {
                    n196 = property on="CameraList 2" class="Ring (严格)"() -> ("StringsAndValues[]"=w206:T2)  [unwired: 2 in, 2 out]
                    n197 = Decrement(x=w204) -> (x-1=w203:u32)
                    n198 = for {
                      N: w203 -> [_]
                      shift-right: [w213] -> w205
                      shift-left: w206 -> [w211]
                      i -> [w208]
                      n199 = Increment(x=w208) -> (x+1=w207:i32)
                      n200 = call "dvp Vi Enum.vi"("unSize"=u32 ?, "index"=w207) -> ("friendlyName out"=w214:string)  [unwired: 8 in, 1 out]
                      n201 = To Unsigned Word Integer(number=w207) -> (unsigned 16bit integer=w210:u16)
                      n202 = Bundle("friendlyName out"=w214, w210) -> (w212:cluster{"friendlyName out":string, u16})  [unwired: 1 in]
                      n203 = Build Array (concatenate)(w211, w212) -> (w213:T2)
                    }
                    n204 = property on="CameraList 2" class="Ring (严格)"("StringsAndValues[]"=w205) -> ()  [unwired: 2 in, 2 out]
                  }
                }
              }
            }
          }
        }
      }
      event #2 {
        w217 = u32 ? items=["OPEN_OFFLINE", "OPEN_NORMAL"] ("type")
        n205 = event-data() -> ()  [unwired: 1 in, 8 out]
        n206 = property on="CameraList 2" class="Ring (严格)"() -> ("RingText.Text"=w216:string)  [unwired: 2 in, 2 out]
        n207 = local write "CloseFlg 2"(i32 ? ("CloseFlg")) -> ()
        n208 = call "dvp Vi Open By Name.vi"("type"=w217, "friendlyName"=w216) -> ("pHandle out"=w219:u32, "function return"=w218:u32)  [unwired: 7 in, 1 out]
        n209 = case shown="1" w218 {
          tunnel: w219 -> [_ w223]
          frame #0 {
            n210 = One Button Dialog(message=string ? ("消息")) -> ()  [unwired: 1 in, 1 out]
          }
          frame #1 {
            n211 = call "dvp Vi Start.vi"("handle"=w223) -> ("function return"=w221:u32)  [unwired: 10 in]
            n212 = local write "handle 2"(w223) -> ()
            n213 = local write "CloseFlg 2"(i32 ? ("CloseFlg")) -> ()
            n214 = case shown="1" w221 {
              tunnel: w223 -> [w226 w228]
              frame #0 {
                w225 = T1 ? ("禁用")
                n215 = local write "CloseFlg 2"(i32 ? ("CloseFlg")) -> ()
                n216 = call "dvp Vi Close.vi"("handle"=w226) -> ()  [unwired: 10 in, 1 out]
                n217 = property on="Set 2" class="Bool"("DisabledEnum"=w225) -> ()  [unwired: 2 in, 2 out]
                n218 = property on="Close 2" class="Bool"("DisabledEnum"=w225) -> ()  [unwired: 2 in, 2 out]
              }
              frame #1 {
                w232 = T1 ? ("禁用")
                n219 = property on="Open 2" class="Bool"("DisabledEnum"=T1 ? ("禁用")) -> ()  [unwired: 2 in, 2 out]
                n220 = call "dvp Vi Get Image Size.vi"("handle"=w228) -> ("function return"=w227:u32)  [unwired: 10 in]
                n221 = Initialize Array(u32 ? ("元素"), w227) -> (w229:u32[])
                n222 = property on="Set 2" class="Bool"("DisabledEnum"=w232) -> ()  [unwired: 2 in, 2 out]
                n223 = property on="Close 2" class="Bool"("DisabledEnum"=w232) -> ()  [unwired: 2 in, 2 out]
                n224 = while {
                  shift-right: [w237] -> _
                  shift-left: w228 -> [w237]
                  tunnel: w229 -> [w238]
                  stop <- w240 stop-if-true
                  n225 = call "dvp Vi Get Image Data.vi"("handle"=w237, "pbuffer"=w238) -> ("piHeight out"=w236:i32, "function return"=w233:bool, "pbuffer out"=w234:u32[], "piWidth out"=w235:i32)  [unwired: 9 in, 1 out]
                  n226 = event shown="[0] \"Close 2\": 鼠标按下" {
                    selector: _ -> [_ _ _]
                    dyn-events: _ -> [_ _ _]
                    timeout: i32 ? -> [_ _ _]
                    tunnel: w237 -> [w242 _ w248]
                    event #0 {
                      n227 = event-data() -> ()  [unwired: 1 in, 5 out]
                      n228 = call "dvp Vi Stop.vi"("handle"=w242) -> ("function return"=w243:u32)  [unwired: 10 in]
                      n229 = case shown="1" w243 {
                        tunnel: w242 -> [_ w245]
                        frame #0 {
                        }
                        frame #1 {
                          w244 = T1 ? ("禁用")
                          n230 = call "dvp Vi Close.vi"("handle"=w245) -> ()  [unwired: 10 in, 1 out]
                          n231 = property on="Open 2" class="Bool"("DisabledEnum"=T1 ? ("禁用")) -> ()  [unwired: 2 in, 2 out]
                          n232 = local write "CloseFlg 2"(i32 ? ("CloseFlg")) -> ()
                          n233 = property on="Close 2" class="Bool"("DisabledEnum"=w244) -> ()  [unwired: 2 in, 2 out]
                          n234 = property on="Set 2" class="Bool"("DisabledEnum"=w244) -> ()  [unwired: 2 in, 2 out]
                        }
                      }
                    }
                    event #1 {
                      n235 = event-data() -> ()  [unwired: 1 in, 3 out]
                    }
                    event #2 {
                      n236 = event-data() -> ()  [unwired: 1 in, 8 out]
                      n237 = call "dvp Vi Show Property Modal Dialog.vi"("handle"=w248) -> ()  [unwired: 10 in, 1 out]
                    }
                  }
                  n238 = case shown="真" w233 {
                    tunnel: w234 -> [_ w252]
                    tunnel: w235 -> [_ w256]
                    tunnel: w236 -> [_ w255]
                    frame #0 {
                    }
                    frame #1 {
                      w272 = u16 ?
                      n239 = property on="new picture 2" class="Pict" props=[]() -> ("Height"=w265:u32, "Width"=w264:u32)  [unwired: 2 in, 3 out]
                      n240 = Type Cast(type=u8[] ?, x=w252) -> (*(type *) &x=w251:u8[])
                      n241 = To Single Precision Float(number=w264) -> (single precision float=w257:sgl)
                      n242 = To Unsigned Word Integer(number=w256) -> (unsigned 16bit integer=w271:u16)
                      n243 = To Unsigned Word Integer(number=w255) -> (unsigned 16bit integer=w270:u16)
                      n244 = To Single Precision Float(number=w265) -> (single precision float=w263:sgl)
                      n245 = To Single Precision Float(number=w256) -> (single precision float=w261:sgl)
                      n246 = To Single Precision Float(number=w255) -> (single precision float=w262:sgl)
                      n247 = Bundle ("图像尺寸")(w272, w272, w271, w270) -> (w269:cluster{u16, u16, u16, u16})  [unwired: 1 in]
                      n248 = Divide(x=w263, y=w262) -> (x/y=w259:sgl)
                      n249 = Divide(x=w257, y=w261) -> (x/y=w258:sgl)
                      n250 = Greater?(x=w259, y=w258) -> (0:w260:bool)
                      n251 = Bundle ("图像数据")("image type"=i16 ?, "image depth"=u8 ?, w251, "无符号8位数组"=u8[] ?, u32[] ?, w269) -> (w253:T3)  [unwired: 1 in]
                      n252 = case shown="真" w260 {
                        tunnel: w259 -> [w275 _]
                        tunnel: w258 -> [_ w276]
                        tunnel: [w275 w276] -> w254
                        frame #0 {
                        }
                        frame #1 {
                        }
                      }
                      n253 = property on="new picture 2" class="Pict"("Erase First"=u8 ? ("画前清除图片")) -> ()  [unwired: 2 in, 2 out]
                      n254 = call <vilib>:"Draw Flattened Pixmap.vi"("image data"=w253) -> ("new picture"=w266:picture)  [unwired: 8 in]
                      n255 = property on="new picture 2" class="Pict"("ZoomFactor"=w254) -> ()  [unwired: 2 in, 2 out]
                      n256 = property on="new picture 2" class="Pict"("Value"=w266) -> ()  [unwired: 2 in, 2 out]
                    }
                  }
                  n257 = local read "CloseFlg 2"() -> (w239:i32)
                  n258 = Equal To 0?(x=w239) -> (x = 0?=w240:bool)
                }
              }
            }
          }
        }
      }
    }
  }
  n259 = while {
    stop <- bool ? stop-if-true
    n260 = event shown="[2] \"Open 4\": 鼠标按下" {
      selector: _ -> [_ _ _]
      dyn-events: _ -> [_ _ _]
      timeout: i32 ? -> [_ _ _]
      event #0 {
        n261 = event-data() -> ()  [unwired: 1 in, 3 out]
      }
      event #1 {
        n262 = event-data() -> ()  [unwired: 1 in, 8 out]
        n263 = stacked-sequence "清除下拉列表的数据" {
          frame #0 {
            n264 = property on="CameraList 4" class="Ring (严格)"() -> ("NumItems"=w279:u32)  [unwired: 2 in, 2 out]
            n265 = for {
              N: w279 -> [_]
              n266 = property on="CameraList 4" class="Ring (严格)"() -> ("Value"=w281:u16)  [unwired: 2 in, 2 out]
              n267 = property on="CameraList 4" class="Ring (严格)"() -> ("Strings []"=w280:string[])  [unwired: 2 in, 2 out]
              n268 = Delete From Array ("删除数组元素")(array=w280, index=w281) -> (array with subset deleted=w282:string[])  [unwired: 1 in, 1 out]
              n269 = property on="CameraList 4" class="Ring (严格)"("Strings []"=w282) -> ()  [unwired: 2 in, 2 out]
            }
          }
          frame #1 {
            n270 = call "dvp Vi Refresh.vi"() -> ("pCount out"=w284:u32)  [unwired: 10 in, 1 out]
            n271 = Greater Than 0?(x=w284) -> (x > 0?=w283:bool)
            n272 = case shown="真" w283 {
              tunnel: w284 -> [_ w285]
              frame #0 {
                # "没有连接的设备直接退出不处理"
              }
              frame #1 {
                n273 = stacked-sequence {
                  tunnel: w285 -> [_ w292]
                  frame #0 {
                    w286 = u32 ? ("index")
                    n274 = property on="CameraList 4" class="Ring (严格)"() -> ("Strings []"=w289:string[])  [unwired: 2 in, 2 out]
                    n275 = call "dvp Vi Enum.vi"("unSize"=u32 ?, "index"=w286) -> ("friendlyName out"=w288:string)  [unwired: 8 in, 1 out]
                    n276 = Replace Array Subset "替换数组子集"(array=w289, new element=w288, index=w286) -> (w290:string[])
                    n277 = property on="CameraList 4" class="Ring (严格)"("Strings []"=w290) -> ()  [unwired: 2 in, 2 out]
                  }
                  frame #1 {
                    n278 = property on="CameraList 4" class="Ring (严格)"() -> ("StringsAndValues[]"=w294:T2)  [unwired: 2 in, 2 out]
                    n279 = Decrement(x=w292) -> (x-1=w291:u32)
                    n280 = for {
                      N: w291 -> [_]
                      shift-right: [w301] -> w293
                      shift-left: w294 -> [w299]
                      i -> [w296]
                      n281 = Increment(x=w296) -> (x+1=w295:i32)
                      n282 = call "dvp Vi Enum.vi"("unSize"=u32 ?, "index"=w295) -> ("friendlyName out"=w302:string)  [unwired: 8 in, 1 out]
                      n283 = To Unsigned Word Integer(number=w295) -> (unsigned 16bit integer=w298:u16)
                      n284 = Bundle("friendlyName out"=w302, w298) -> (w300:cluster{"friendlyName out":string, u16})  [unwired: 1 in]
                      n285 = Build Array (concatenate)(w299, w300) -> (w301:T2)
                    }
                    n286 = property on="CameraList 4" class="Ring (严格)"("StringsAndValues[]"=w293) -> ()  [unwired: 2 in, 2 out]
                  }
                }
              }
            }
          }
        }
      }
      event #2 {
        w305 = u32 ? items=["OPEN_OFFLINE", "OPEN_NORMAL"] ("type")
        n287 = event-data() -> ()  [unwired: 1 in, 8 out]
        n288 = property on="CameraList 4" class="Ring (严格)"() -> ("RingText.Text"=w304:string)  [unwired: 2 in, 2 out]
        n289 = local write "CloseFlg 4"(i32 ? ("CloseFlg")) -> ()
        n290 = call "dvp Vi Open By Name.vi"("type"=w305, "friendlyName"=w304) -> ("pHandle out"=w307:u32, "function return"=w306:u32)  [unwired: 7 in, 1 out]
        n291 = case shown="1" w306 {
          tunnel: w307 -> [_ w311]
          frame #0 {
            n292 = One Button Dialog(message=string ? ("消息")) -> ()  [unwired: 1 in, 1 out]
          }
          frame #1 {
            n293 = call "dvp Vi Start.vi"("handle"=w311) -> ("function return"=w309:u32)  [unwired: 10 in]
            n294 = local write "handle 4"(w311) -> ()
            n295 = local write "CloseFlg 4"(i32 ? ("CloseFlg")) -> ()
            n296 = case shown="1" w309 {
              tunnel: w311 -> [w314 w316]
              frame #0 {
                w313 = T1 ? ("禁用")
                n297 = local write "CloseFlg 4"(i32 ? ("CloseFlg")) -> ()
                n298 = call "dvp Vi Close.vi"("handle"=w314) -> ()  [unwired: 10 in, 1 out]
                n299 = property on="Set 4" class="Bool"("DisabledEnum"=w313) -> ()  [unwired: 2 in, 2 out]
                n300 = property on="Close 4" class="Bool"("DisabledEnum"=w313) -> ()  [unwired: 2 in, 2 out]
              }
              frame #1 {
                w320 = T1 ? ("禁用")
                n301 = property on="Open 4" class="Bool"("DisabledEnum"=T1 ? ("禁用")) -> ()  [unwired: 2 in, 2 out]
                n302 = call "dvp Vi Get Image Size.vi"("handle"=w316) -> ("function return"=w315:u32)  [unwired: 10 in]
                n303 = Initialize Array(u32 ? ("元素"), w315) -> (w317:u32[])
                n304 = property on="Set 4" class="Bool"("DisabledEnum"=w320) -> ()  [unwired: 2 in, 2 out]
                n305 = property on="Close 4" class="Bool"("DisabledEnum"=w320) -> ()  [unwired: 2 in, 2 out]
                n306 = while {
                  shift-right: [w325] -> _
                  shift-left: w316 -> [w325]
                  tunnel: w317 -> [w326]
                  stop <- w328 stop-if-true
                  n307 = call "dvp Vi Get Image Data.vi"("handle"=w325, "pbuffer"=w326) -> ("piHeight out"=w324:i32, "function return"=w321:bool, "pbuffer out"=w322:u32[], "piWidth out"=w323:i32)  [unwired: 9 in, 1 out]
                  n308 = event shown="[1] 超时" {
                    selector: _ -> [_ _ _]
                    dyn-events: _ -> [_ _ _]
                    timeout: i32 ? -> [_ _ _]
                    tunnel: w325 -> [w330 _ w336]
                    event #0 {
                      n309 = event-data() -> ()  [unwired: 1 in, 5 out]
                      n310 = call "dvp Vi Stop.vi"("handle"=w330) -> ("function return"=w331:u32)  [unwired: 10 in]
                      n311 = case shown="1" w331 {
                        tunnel: w330 -> [_ w333]
                        frame #0 {
                        }
                        frame #1 {
                          w332 = T1 ? ("禁用")
                          n312 = call "dvp Vi Close.vi"("handle"=w333) -> ()  [unwired: 10 in, 1 out]
                          n313 = property on="Open 4" class="Bool"("DisabledEnum"=T1 ? ("禁用")) -> ()  [unwired: 2 in, 2 out]
                          n314 = local write "CloseFlg 4"(i32 ? ("CloseFlg")) -> ()
                          n315 = property on="Close 4" class="Bool"("DisabledEnum"=w332) -> ()  [unwired: 2 in, 2 out]
                          n316 = property on="Set 4" class="Bool"("DisabledEnum"=w332) -> ()  [unwired: 2 in, 2 out]
                        }
                      }
                    }
                    event #1 {
                      n317 = event-data() -> ()  [unwired: 1 in, 3 out]
                    }
                    event #2 {
                      n318 = event-data() -> ()  [unwired: 1 in, 8 out]
                      n319 = call "dvp Vi Show Property Modal Dialog.vi"("handle"=w336) -> ()  [unwired: 10 in, 1 out]
                    }
                  }
                  n320 = case shown="真" w321 {
                    tunnel: w322 -> [_ w340]
                    tunnel: w323 -> [_ w344]
                    tunnel: w324 -> [_ w343]
                    frame #0 {
                    }
                    frame #1 {
                      w360 = u16 ?
                      n321 = property on="new picture 4" class="Pict" props=[]() -> ("Height"=w353:u32, "Width"=w352:u32)  [unwired: 2 in, 3 out]
                      n322 = Type Cast(type=u8[] ?, x=w340) -> (*(type *) &x=w339:u8[])
                      n323 = To Single Precision Float(number=w352) -> (single precision float=w345:sgl)
                      n324 = To Unsigned Word Integer(number=w344) -> (unsigned 16bit integer=w359:u16)
                      n325 = To Unsigned Word Integer(number=w343) -> (unsigned 16bit integer=w358:u16)
                      n326 = To Single Precision Float(number=w353) -> (single precision float=w351:sgl)
                      n327 = To Single Precision Float(number=w344) -> (single precision float=w349:sgl)
                      n328 = To Single Precision Float(number=w343) -> (single precision float=w350:sgl)
                      n329 = Bundle ("图像尺寸")(w360, w360, w359, w358) -> (w357:cluster{u16, u16, u16, u16})  [unwired: 1 in]
                      n330 = Divide(x=w351, y=w350) -> (x/y=w347:sgl)
                      n331 = Divide(x=w345, y=w349) -> (x/y=w346:sgl)
                      n332 = Greater?(x=w347, y=w346) -> (0:w348:bool)
                      n333 = Bundle ("图像数据")("image type"=i16 ?, "image depth"=u8 ?, w339, "无符号8位数组"=u8[] ?, u32[] ?, w357) -> (w341:T3)  [unwired: 1 in]
                      n334 = case shown="真" w348 {
                        tunnel: w347 -> [w363 _]
                        tunnel: w346 -> [_ w364]
                        tunnel: [w363 w364] -> w342
                        frame #0 {
                        }
                        frame #1 {
                        }
                      }
                      n335 = property on="new picture 4" class="Pict"("Erase First"=u8 ? ("画前清除图片")) -> ()  [unwired: 2 in, 2 out]
                      n336 = call <vilib>:"Draw Flattened Pixmap.vi"("image data"=w341) -> ("new picture"=w354:picture)  [unwired: 8 in]
                      n337 = property on="new picture 4" class="Pict"("ZoomFactor"=w342) -> ()  [unwired: 2 in, 2 out]
                      n338 = property on="new picture 4" class="Pict"("Value"=w354) -> ()  [unwired: 2 in, 2 out]
                    }
                  }
                  n339 = local read "CloseFlg 4"() -> (w327:i32)
                  n340 = Equal To 0?(x=w327) -> (x = 0?=w328:bool)
                }
              }
            }
          }
        }
      }
    }
  }
  "handle" <- u32 ? ("handle")
  "handle 2" <- u32 ? ("handle")
  "handle 3" <- u32 ? ("handle")
  "handle 4" <- u32 ? ("handle")
